vi "Get Configuration.vi"(6 "timeout (ms)":i32=5000, 8 "error in":errorcluster, 11 "gRPC ID":T1) -> (0 "error out":errorcluster, 2 "JSON Configuration":string, 3 "gRPC ID out":T1)   [LabVIEW 2021, in "CIFCoreWrapper.lvlib"]
uses:
  CIFCoreWrapper.lvlib
  <vilib>/gRPC/LabVIEW gRPC Library/Shared/grpcId.ctl
  CIFCorePlugin_client/CIFCorePlugin_client.lvlib
  <vilib>/gRPC/LabVIEW gRPC Library/grpc-lvsupport-release.lvlib
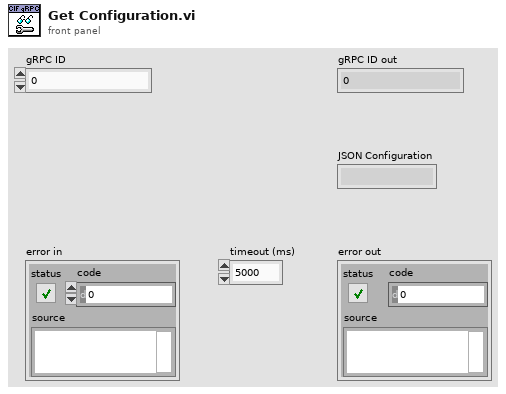
[diagram p1: front panel]
types:
  T1 = typedef "grpc-lvsupport-release.lvlib/grpcId.ctl" = u64
  T2 = typedef "CIFCorePlugin_client.lvlib/cif_plugincore_Configuration.ctl" = cluster{"json_config":string}
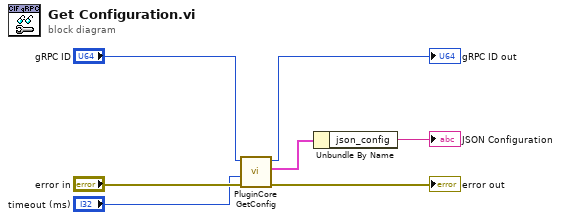
[diagram p0: block diagram]
diagram:
  n1 = call "PluginCore GetConfig.vi"("error in"="error in", "timeout (ms)"="timeout (ms)", "gRPC ID"="gRPC ID") -> ("error out"=→"error out":errorcluster, "Response Data"=w3:T2, "gRPC ID out"=→"gRPC ID out":T1)  [unwired: 6 in]
  n2 = Unbundle By Name(w3) -> ("json_config"=→"JSON Configuration":string)
